vi "Goto.vi"(6 "Home?":bool, 7 "Speed":i32, 8 "error in (no error)":errorcluster, 9 "channel":i32(ring)=1 items=["Channel1"=1, "Channel2"=2, "Channel3"=3, "Channel4"=4], 10 "New Position":sgl, 11 "TranslationStage in":refnum<class "ArduinoTranslationStage.lvclass">) -> (0 "error out":errorcluster, 3 "TranslationStage out":refnum<class "ArduinoTranslationStage.lvclass">)   [LabVIEW 2023, in "TranslationStage Library.lvlib" / "ArduinoTranslationStage.lvlib" / "ArduinoTranslationStage.lvclass"]
uses:
  ArduinoTranslationStage.lvclass
  ArduinoTranslationStage.lvclass/ArduinoTranslationStage.ctl
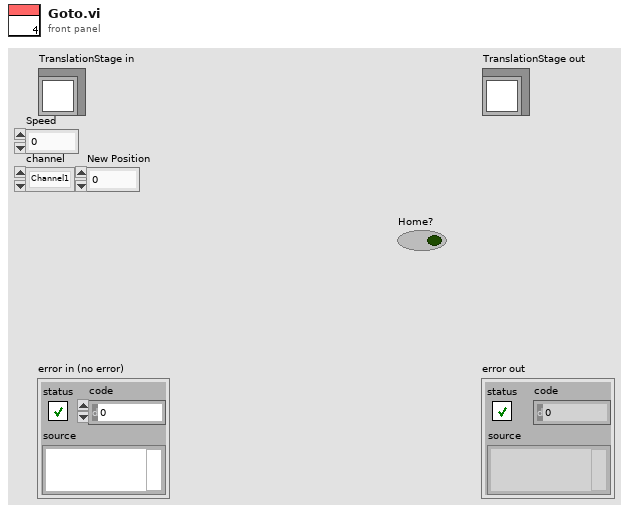
[diagram p1: front panel]
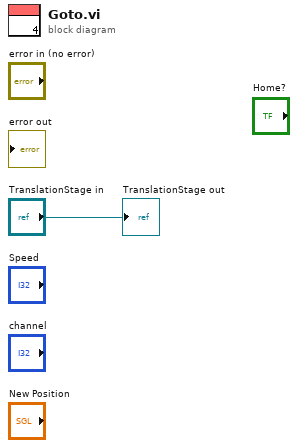
[diagram p0: block diagram]
diagram:
  "TranslationStage out" <- "TranslationStage in"
